vi "User_Add.vi"() -> (2 "Ok？":bool)   [LabVIEW 2020]
panel:
  in  "User_Right":u16(ring) caption="权        限" items=["管理员", "操作员"]
  in  "Confirm Password":string caption="确认密码"
  in  "New Password":string caption="密        码"
  in  "Ok":bool
  in  "User_Name":string caption="用  户  名"
  # "添加用户"
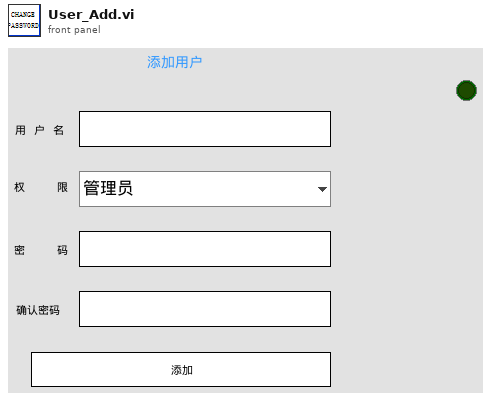
[diagram p1: front panel]
types:
  T1 = enum8{"Enabled", "Disabled", "Disabled and Grayed Out"}
  T2 = typedef "User_Info.ctl" = cluster{"Name":string, "Password":string, "User_Right":u16, "Debuger?":bool, "Manager?":bool, "User_Remember_Name":bool, "User_Remember_PW":bool, "User_Right_String":string, "Null?":bool, "Language":string}
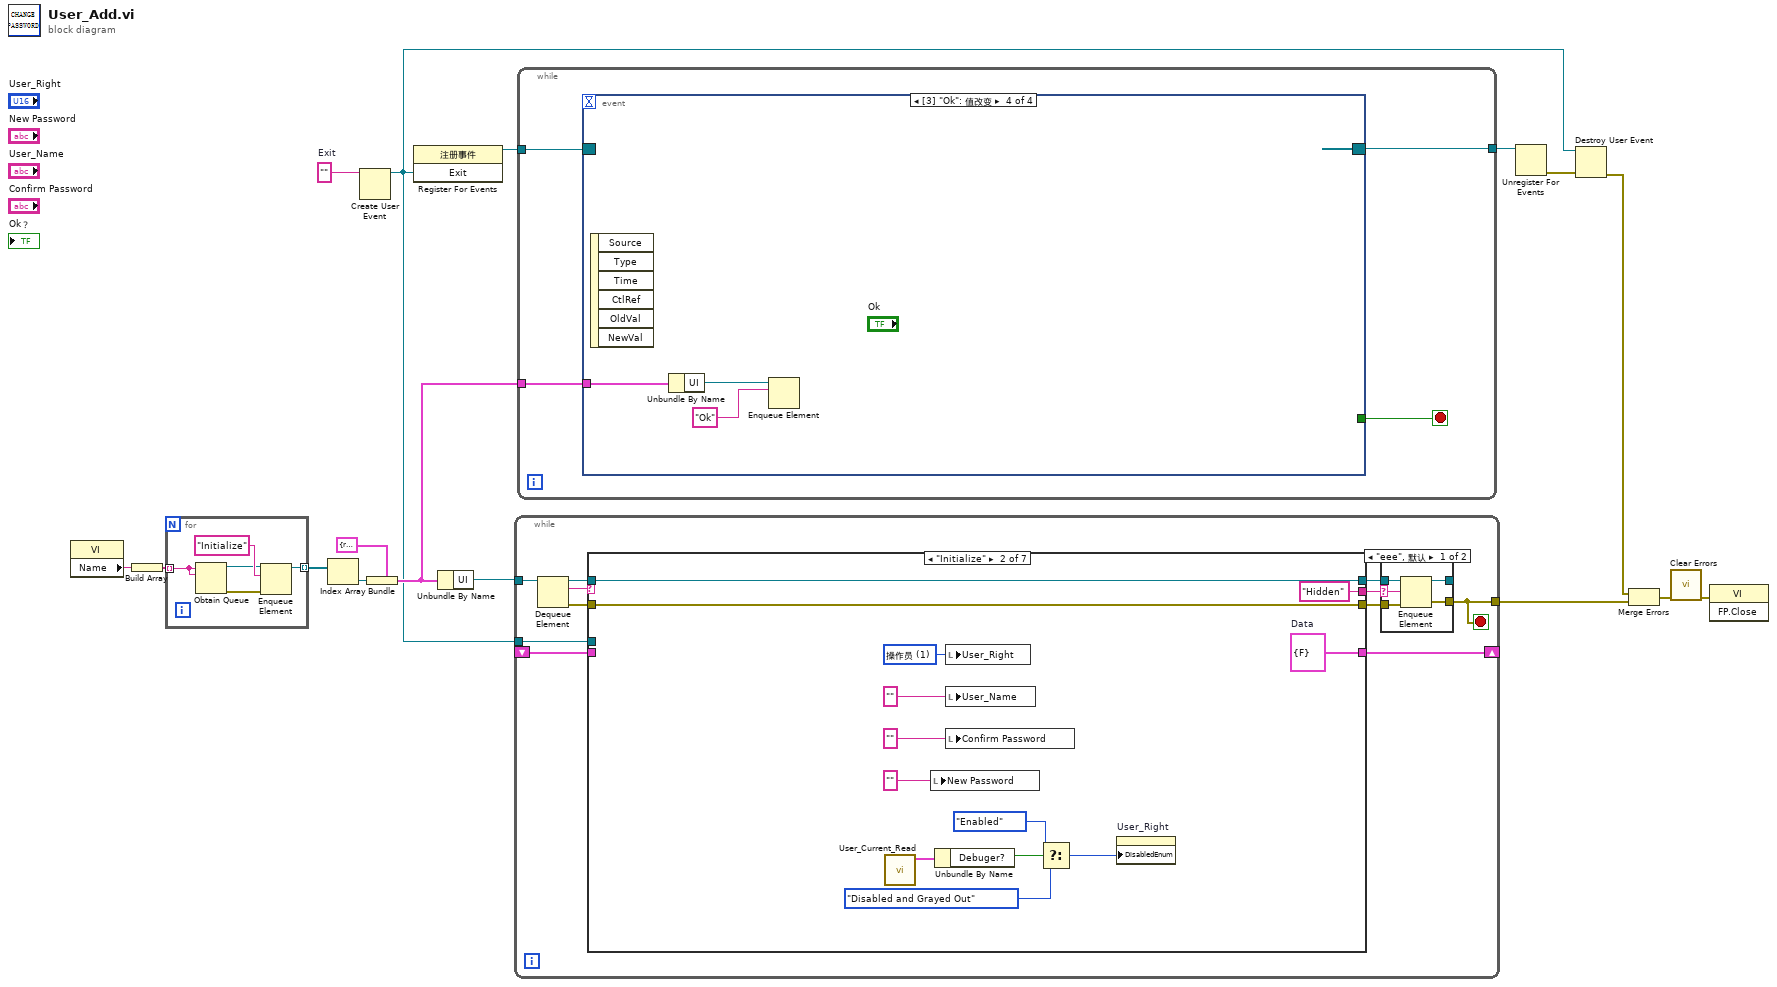
[diagram p0: block diagram]
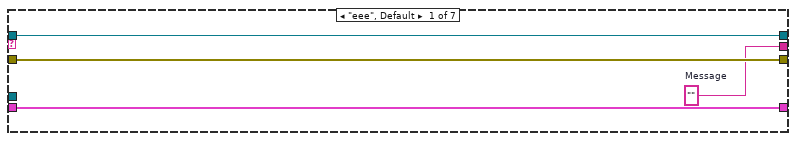
[diagram p3: hidden frame]
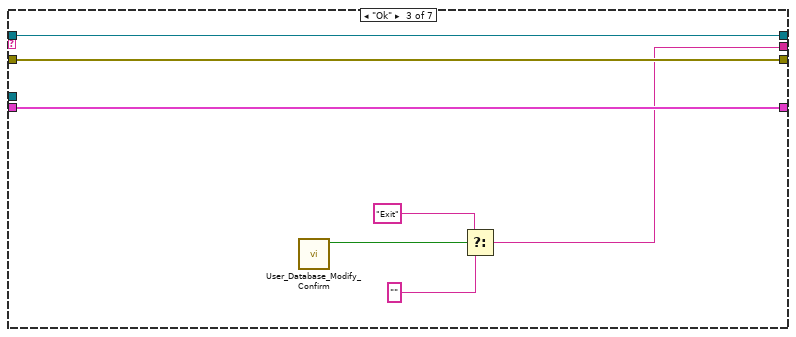
[diagram p4: hidden frame]
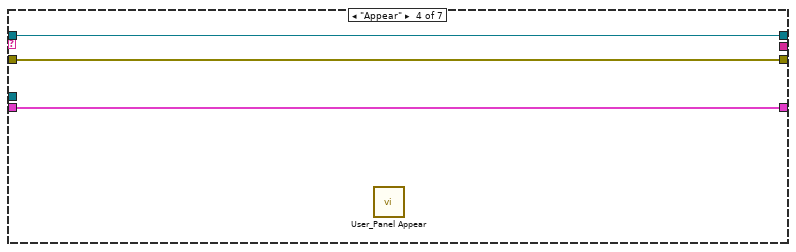
[diagram p5: hidden frame]
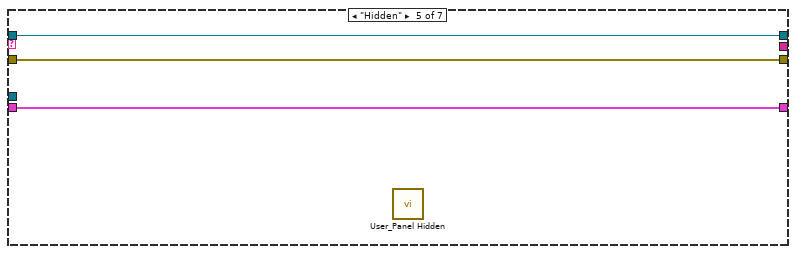
[diagram p6: hidden frame]
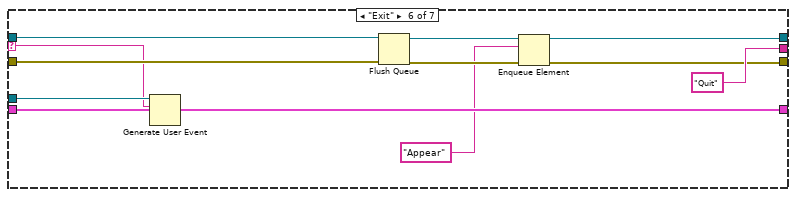
[diagram p7: hidden frame]
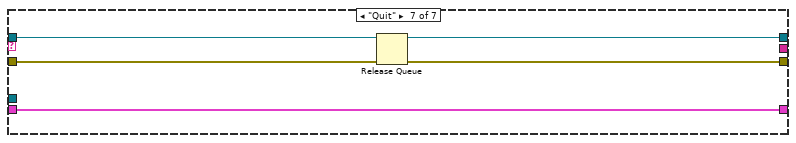
[diagram p8: hidden frame]
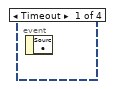
[diagram p9: hidden frame]
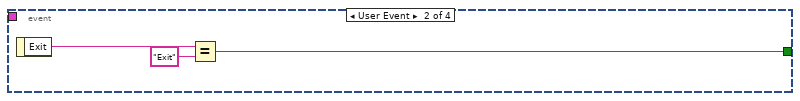
[diagram p10: hidden frame]
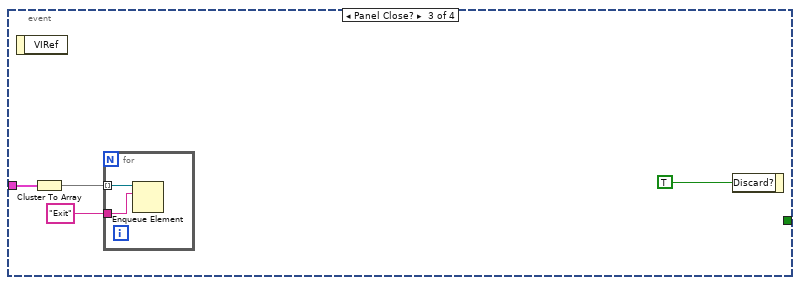
[diagram p11: hidden frame]
diagram:
  w2 = ""  # Exit
  n1 = property class="VI"() -> ("Name"=w12:string)  [unwired: 2 in, 2 out]
  n2 = Build Array(w12) -> (w13:string[])
  n3 = for {
    tunnel: w13 -> [w17] mode=indexing
    tunnel: [w18] -> w7 mode=indexing
    n4 = Obtain Queue(name (unnamed)=w17, element data type=w17) -> (queue out=w20:refnum<queue>, error out=w19:errorcluster)  [unwired: 3 in, 1 out]
    n5 = Enqueue Element(queue=w20, element="Initialize" ("元素"), error in (no error)=w19) -> (queue out=w18:refnum<queue>)  [unwired: 1 in, 2 out]
  }
  n6 = Index Array(array=w7) -> (element=w10:refnum<queue>)  [unwired: 1 in]
  n7 = Create User Event(user event datatype=w2) -> (user event=w6:refnum<user-event>)  [unwired: 1 in, 1 out]
  n8 = Bundle(cluster=cluster{"UI":refnum<queue>} {"UI"=refnum}, "UI"=w10) -> (w11:cluster{"UI":refnum<queue>})
  n9 = register-events(w6) -> (reference out=w3:refnum<event-registration>)  [unwired: 2 in, 1 out]
  n10 = Unbundle By Name(w11) -> ("UI"=w8:refnum<queue>)
  n11 = while {
    tunnel: w8 -> [w32]
    tunnel: [w22] -> w15
    shift-right: [w26] -> _
    shift-left: _ -> [w25]
    tunnel: w6 -> [w24]
    stop <- w22 stop-if-true
    n12 = Dequeue Element(queue=w32) -> (queue out=w31:refnum<queue>, element=w23:string, error out=w28:errorcluster)  [unwired: 2 in, 1 out]
    n13 = case shown="\"Initialize\"" w23 {
      selector: w23 -> [_ _ _ _ _ w75 _]
      tunnel: w31 -> [w43 w56 w63 w66 w69 w78 w84]
      tunnel: [w43 w56 w63 w66 w69 w73 w84] -> w30
      tunnel: [w42 w55 w62 w65 w68 w71 w81] -> w29
      tunnel: w28 -> [w42 w55 w62 w65 w68 w77 w83]
      tunnel: [w41 "Hidden" ("Message") w57 _ _ "Quit" ("Message") _] -> w27
      tunnel: [w40 w54 w61 w64 w67 w80 w82] -> w26
      tunnel: w25 -> [w40 _ w61 w64 w67 w80 w82]
      tunnel: w24 -> [_ _ _ _ _ w76 _]
      frame "eee", Default {
        w41 = ""  # Message
      }
      frame "Initialize" {
        w53 = u16 1 items=["管理员", "操作员"] ("User_Right")
        w54 = cluster{"Data":bool} {"Data"=FALSE}  # Data
        n14 = call "User_Current_Read.vi"() -> ("User_Info"=w48:T2)  [unwired: 10 in, 1 out]
        n15 = local write "New Password"("" ("Password")) -> ()
        n16 = Unbundle By Name(w48) -> ("Debuger?"=w47:bool)
        n17 = local write "User_Right"(w53) -> ()
        n18 = local write "User_Name"("" ("User_Name")) -> ()
        n19 = local write "Confirm Password"("" ("Confirm Password")) -> ()
        n20 = Select(t=T1."Enabled" ("禁用"), s=w47, f=T1."Disabled and Grayed Out" ("禁用")) -> (s? t:f=w45:T1)
        n21 = property on="User_Right" class="Ring (严格)"("DisabledEnum"=w45) -> ()  [unwired: 2 in, 2 out]
      }
      frame "Ok" {
        n22 = call "User_Database_Modify_Confirm.vi"() -> ("OK"=w60:bool)  [unwired: 10 in, 1 out]
        n23 = Select(t="Exit", s=w60, f="") -> (s? t:f=w57:string)
      }
      frame "Appear" {
        n24 = call "User_Panel Appear.vi"() -> ()  [unwired: 11 in, 1 out]
      }
      frame "Hidden" {
        n25 = call "User_Panel Hidden.vi"() -> ()  [unwired: 11 in, 1 out]
      }
      frame "Exit" {
        n26 = Generate User Event(user event=w76, event data cluster=w75) -> ()  [unwired: 2 in, 2 out]
        n27 = Flush Queue(queue=w78, error in (no error)=w77) -> (queue out=w74:refnum<queue>, error out=w72:errorcluster)  [unwired: 1 out]
        n28 = Enqueue Element(queue=w74, element="Appear" ("元素"), error in (no error)=w72) -> (queue out=w73:refnum<queue>, error out=w71:errorcluster)  [unwired: 1 in, 1 out]
      }
      frame "Quit" {
        n29 = Release Queue(queue=w84, error in (no error)=w83) -> (error out=w81:errorcluster)  [unwired: 1 in, 2 out]
      }
    }
    n30 = case shown="\"eee\", 默认" w27 {
      selector: w27 -> [w33 _]
      tunnel: w30 -> [w37 w39]
      tunnel: w29 -> [w36 w38]
      tunnel: [w35 w38] -> w22
      tunnel: [w34 w39] -> _
      frame "eee", Default {
        n31 = Enqueue Element(queue=w37, element=w33, error in (no error)=w36) -> (queue out=w34:refnum<queue>, error out=w35:errorcluster)  [unwired: 1 in, 1 out]
      }
      frame "" {
      }
    }
  }
  n32 = while {
    tunnel: w3 -> [w87]
    tunnel: [w86] -> w5
    tunnel: w11 -> [w85]
    stop <- w88 stop-if-true
    n33 = event shown="[3] \"Ok\": 值改变" {
      selector: w87 -> [_ _ _ _]
      dyn-events: [_ _ _ _] -> w86
      timeout: _ -> [_ _ _ _]
      tunnel: [_ w90 _ _] -> w88
      tunnel: w85 -> [_ _ w94 w100]
      event Timeout {
        n34 = event-data() -> ()  [unwired: 1 in, 1 out]
      }
      event User Event {
        n35 = event-data() -> ("Exit"=w91:string)  [unwired: 1 in]
        n36 = Equal?(x=w91, y="Exit") -> (x = y?=w90:bool)
      }
      event Panel Close? {
        n37 = event-data() -> ()  [unwired: 1 in, 1 out]
        n38 = Cluster To Array(cluster=w94) -> (array=w93:refnum<queue>[])
        n39 = for {
          tunnel: w93 -> [w97] mode=indexing
          tunnel: "Exit" ("元素") -> [w96]
          n40 = Enqueue Element(queue=w97, element=w96) -> ()  [unwired: 2 in, 3 out]
        }
        n41 = event-data("Discard?"=TRUE ("放弃？")) -> ()  [unwired: 1 in, 1 out]
      }
      event "Ok": Value Change {
        n42 = event-data() -> ()  [unwired: 1 in, 6 out]
        n43 = Unbundle By Name(w100) -> ("UI"=w99:refnum<queue>)
        n44 = Enqueue Element(queue=w99, element="Ok" ("元素")) -> ()  [unwired: 2 in, 3 out]
      }
    }
  }
  n45 = Unregister For Events(event registration refnum=w5) -> (error out=w4:errorcluster)  [unwired: 1 in]
  n46 = Destroy User Event(user event=w6, error in=w4) -> (error out=w14:errorcluster)
  n47 = Merge Errors(w14, w15) -> (w16:errorcluster)
  n48 = call <vilib>:"Clear Errors.vi"("error in (no error)"=w16) -> ("error out"=w1:errorcluster)  [unwired: 5 in, 1 out]
  n49 = invoke class="VI" method="FP.Close"(error in=w1) -> ()  [unwired: 2 in, 3 out]
